vi "数据采集1channel.vi"() -> ()   [LabVIEW 2018]
panel:
  in  "File Name":string
  in  "File Path":path
  in  "stop (F)":bool caption="停止(F)"
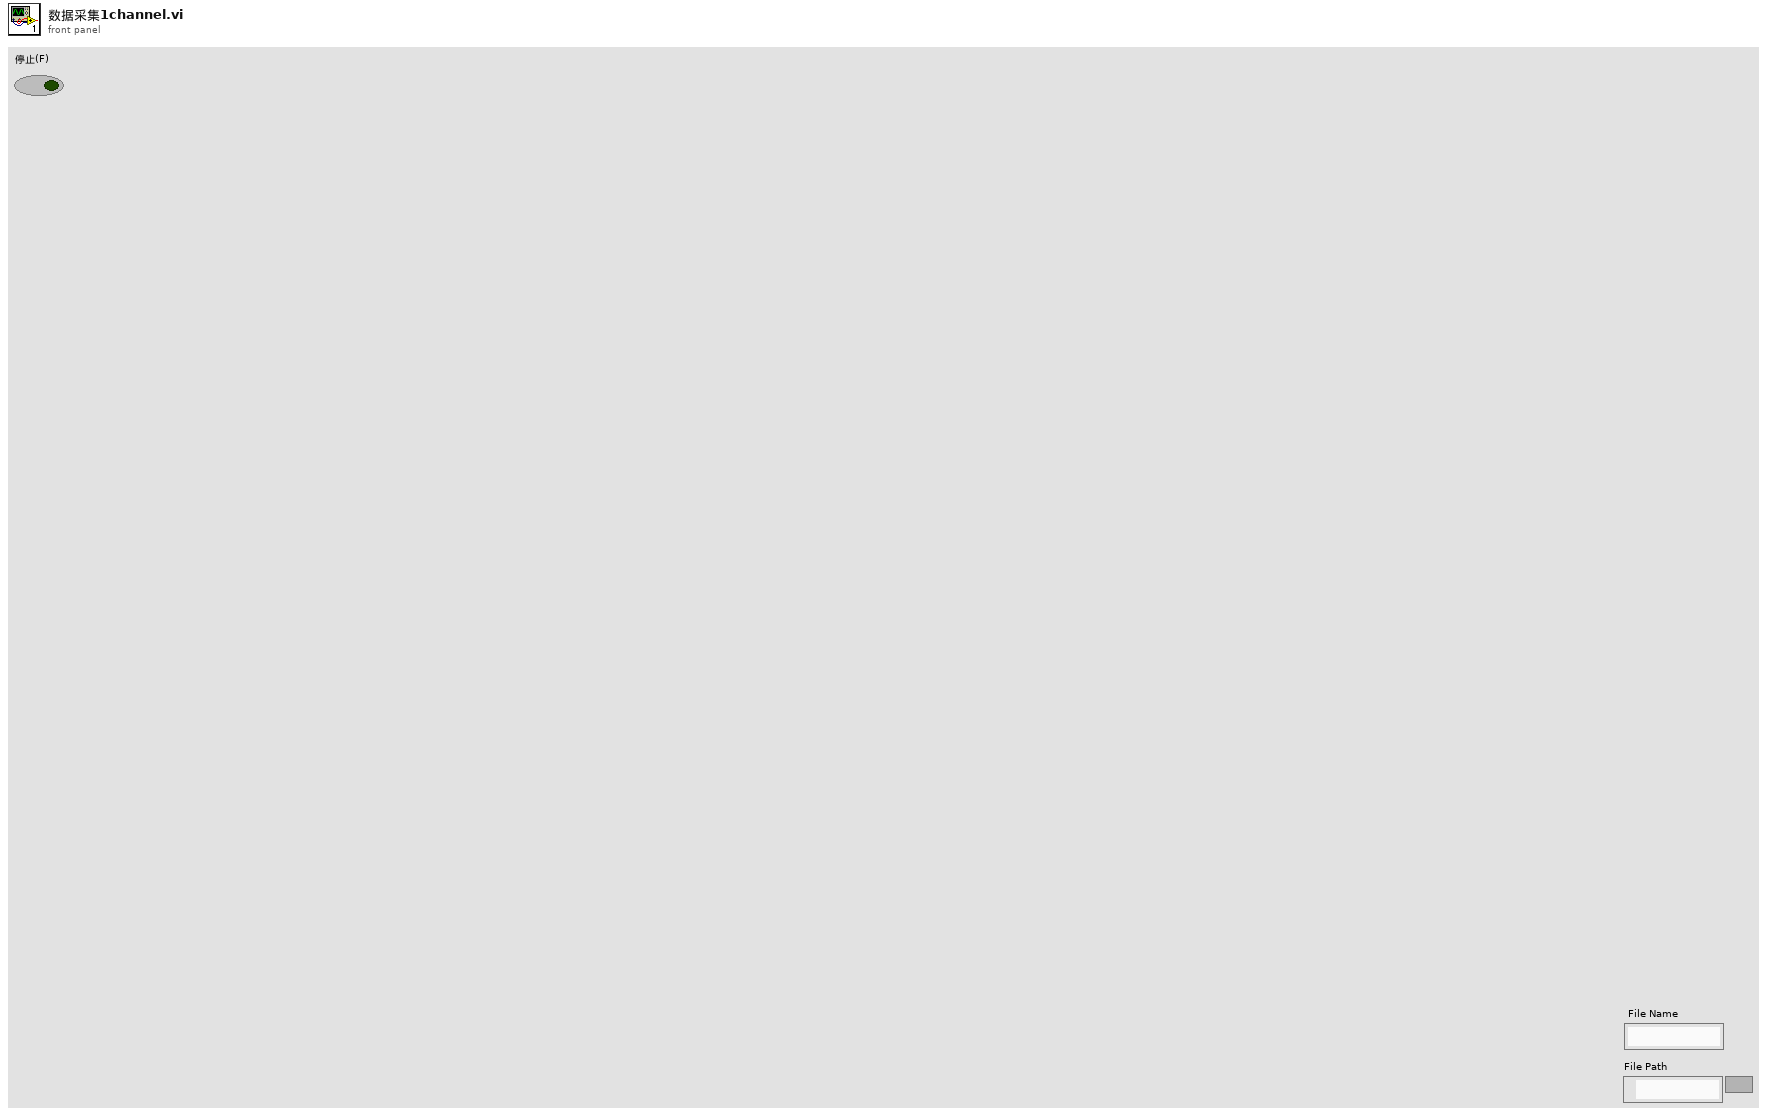
[diagram p1: front panel]
types:
  T1 = enum16{"open", "replace", "create", "open or create", "replace or create", "replace or create with confirmation"}
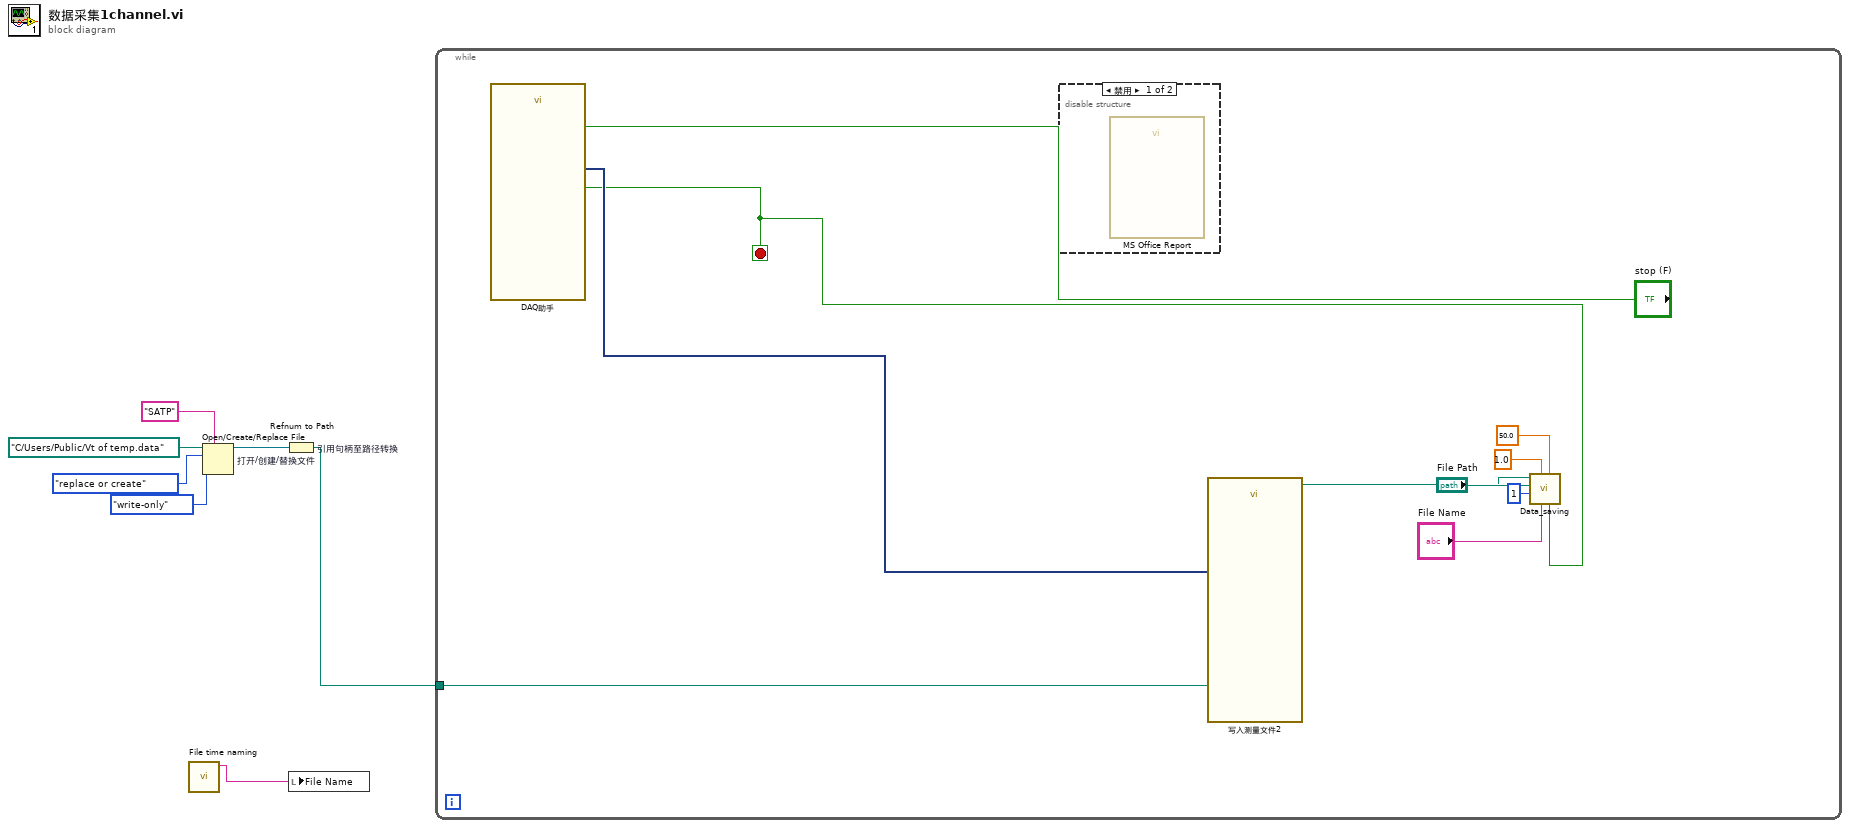
[diagram p0: block diagram]
diagram:
  n1 = call "File time naming.vi"() -> ("result string"=w7:string)  [unwired: 11 in]
  n2 = Open/Create/Replace File "打开/创建/替换文件"(file path (use dialog)=path "C:/Users/Public/Vt of temp.data" ("文件路径（使用对话框）"), prompt="SATP" ("提示"), operation (0:open)=T1."replace or create" ("操作(0:open)"), access (0:read/write)=enum16{"read/write", "read-only", "write-only"}."write-only" ("权限(0:read/write)")) -> (refnum out=w3:refnum<file>)  [unwired: 2 in, 2 out]
  n3 = Refnum to Path "引用句柄至路径转换"(1:w3) -> (0:w1:path)
  n4 = local write "File Name"(w7) -> ()
  n5 = while {
    tunnel: w1 -> [w10]
    stop <- w8 stop-if-true
    n6 = call "DAQ助手"("stop (F)"="stop (F)") -> ("data"=w11:dynamicdata, "stopped"=w8:bool)  [unwired: 15 in, 2 out]
    n7 = disable-structure shown="禁用" {
      frame Disabled {
        n8 = call "MS Office Report"() -> ()  [unwired: 27 in, 1 out]
      }
      frame Enabled {
      }
    }
    n9 = call "写入测量文件2"("Signals"=w11, "Filename"=w10) -> ("Filename Out"=w12:path)  [unwired: 15 in, 2 out]
    n10 = call "Data_saving.vi"("Boolean"=w8, "Sampling Rate"=50.0, "File Name"="File Name", "Voltage Sensitivity\n1000 will be 1000"=1.0 ("Voltage Sensitivity\n1000 will be 1000"), "Number of Samples Per Channel"=1, "File Path"="File Path", "File name source"=w12) -> ()  [unwired: 5 in]
  }
